vi "Create Event.vi"(9 "Event jettl":refnum<class "Event jettl.lvclass">, 10 "Alias":string, 11 "Base Queue jettl in":refnum<class "Base Queue jettl.lvclass">) -> (3 "Base Queue jettl out":refnum<class "Base Queue jettl.lvclass">)   [LabVIEW 2021, in "jettl.lvlib" / "Base Queue jettl.lvlib" / "Base Queue jettl.lvclass"]
uses:
  Base Queue jettl.lvclass
  Event jettl/Event jettl.lvclass
  Msg Strategy/Msg Strategy.lvclass
  Base Queue jettl.lvclass/Base Queue jettl.ctl
  jettl.lvlib
  Queue Mailbox/Queue Mailbox.lvlib
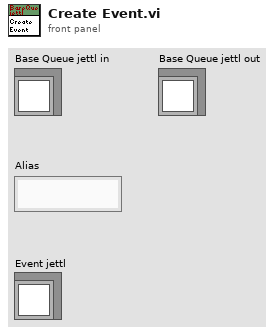
[diagram p1: front panel]
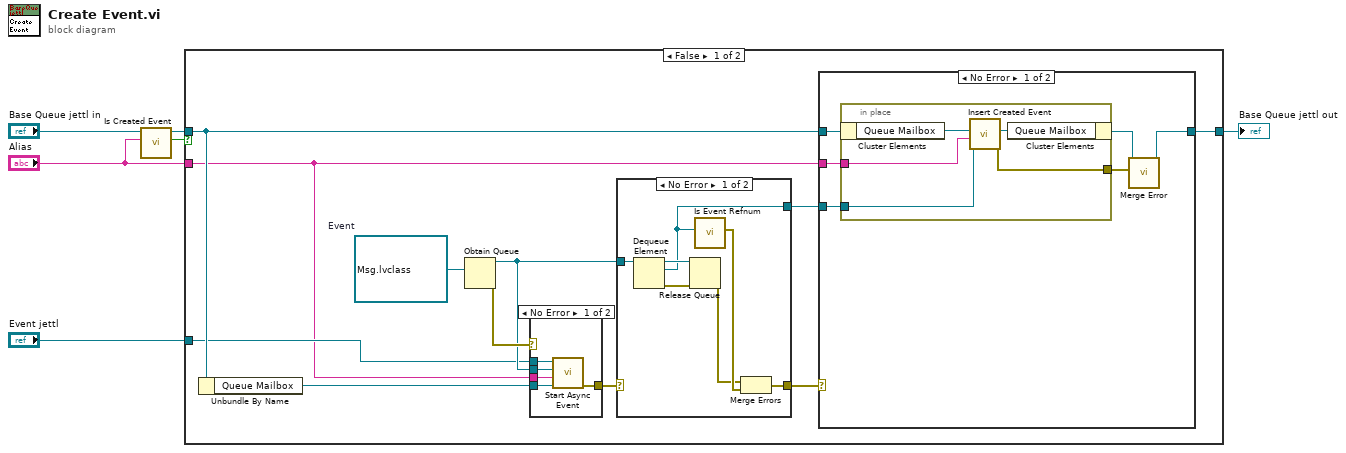
[diagram p0: block diagram]
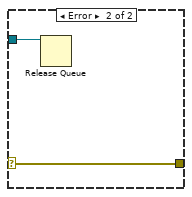
[diagram p2: hidden frame]
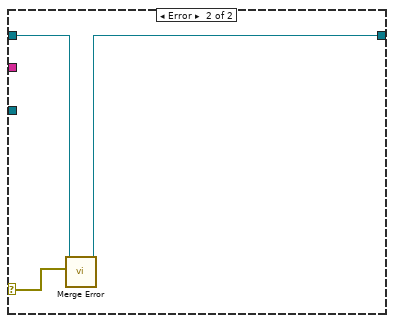
[diagram p4: hidden frame]
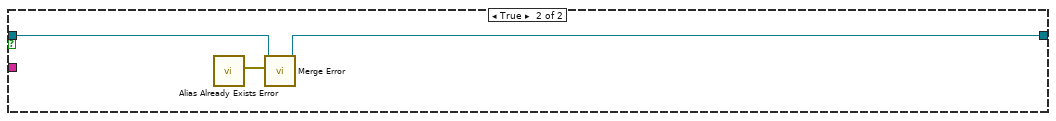
[diagram p5: hidden frame]
diagram:
  n1 = call-dynamic "Is Created Event.vi"("Created Event Alias"="Alias", "Base Queue jettl in"="Base Queue jettl in") -> ("Is Created Event?"=w2:bool, "Base Queue jettl out"=w1:refnum<class "Base Queue jettl.lvclass">)  [unwired: 8 in]
  n2 = case shown="False" w2 {
    tunnel: "Event jettl" -> [w12 _]
    tunnel: w1 -> [w15 w49]
    tunnel: "Alias" -> [w7 _]
    tunnel: [w14 w48] -> w5
    frame False {
      w9 = refnum<data-value> refnum  # Event
      n3 = Unbundle By Name(w15) -> ("Queue Mailbox"=w8:refnum<data-value>)
      n4 = Obtain Queue(element data type=w9) -> (queue out=w13:refnum<queue>, error out=w17:errorcluster)  [unwired: 4 in, 1 out]
      n5 = case shown="No Error" w17 {
        selector: w17 -> [_ w32]
        tunnel: [w30 w32] -> w10
        tunnel: w12 -> [w31 _]
        tunnel: w13 -> [w28 _]
        tunnel: w7 -> [w27 _]
        tunnel: w8 -> [w29 _]
        frame No Error {
          n6 = call "Start Async Event.vi"("Queue Mailbox"=w29, "Self Alias"=w27, "Queue of Event Self"=w28, "Event jettl"=w31) -> ("error out"=w30:errorcluster)  [unwired: 7 in]
        }
        frame Error {
        }
      }
      n7 = case shown="No Error" w10 {
        selector: w10 -> [_ w26]
        tunnel: [w22 w26] -> w16
        tunnel: w13 -> [w21 w25]
        tunnel: [w20 _] -> w11
        frame No Error {
          n8 = Dequeue Element(queue=w21) -> (queue out=w23:refnum<queue>, element=w20:refnum<data-value>, error out=w24:errorcluster)  [unwired: 2 in, 1 out]
          n9 = Release Queue(queue=w23, error in (no error)=w24) -> (error out=w18:errorcluster)  [unwired: 1 in, 2 out]
          n10 = call "Is Event Refnum.vi"("Event"=w20) -> ("Error"=w19:errorcluster)  [unwired: 10 in]
          n11 = Merge Errors(w18, w19) -> (w22:errorcluster)
        }
        frame Error {
          n12 = Release Queue(queue=w25) -> ()  [unwired: 2 in, 3 out]
        }
      }
      n13 = case shown="No Error" w16 {
        selector: w16 -> [_ w44]
        tunnel: w15 -> [w38 w46]
        tunnel: [w34 w45] -> w14
        tunnel: w11 -> [w37 _]
        tunnel: w7 -> [w36 _]
        frame No Error {
          n14 = in-place {
            in-place-border: w37 -> [w40]
            in-place-border: w36 -> [w41]
            in-place-border: [w39] -> w33
            n15 = in-place-cluster #1(w38) -> ("Queue Mailbox"=w43:refnum<data-value>)
            n16 = call "Insert Created Event.vi"("Self Event"=w40, "Self Event Alias"=w41, "Queue Mailbox in"=w43) -> ("error out"=w39:errorcluster, "Queue Mailbox out"=w42:refnum<data-value>)  [unwired: 7 in]
            n17 = in-place-cluster #1("Queue Mailbox"=w42) -> (w35:refnum<class "Base Queue jettl.lvclass">)
          }
          n18 = call-dynamic "Merge Error.vi"("Error"=w33, "Base Queue jettl in"=w35) -> ("Base Queue jettl out"=w34:refnum<class "Base Queue jettl.lvclass">)  [unwired: 9 in]
        }
        frame Error {
          n19 = call-dynamic "Merge Error.vi"("Error"=w44, "Base Queue jettl in"=w46) -> ("Base Queue jettl out"=w45:refnum<class "Base Queue jettl.lvclass">)  [unwired: 9 in]
        }
      }
    }
    frame True {
      n20 = call "Alias Already Exists Error.vi"() -> ("Error"=w47:errorcluster)  [unwired: 11 in]
      n21 = call-dynamic "Merge Error.vi"("Error"=w47, "Base Queue jettl in"=w49) -> ("Base Queue jettl out"=w48:refnum<class "Base Queue jettl.lvclass">)  [unwired: 9 in]
    }
  }
  "Base Queue jettl out" <- w5
